vi "M9290A Configure Sweep.vi"(4 "Manual Mechanical Attenuation (10 dB)":dbl=10.0, 6 "Trigger Level":dbl=20.0, 7 "Trigger Source (0: Free Run)":i32(ring) items=["Free Run", "Video", "Line", "External1", "External2", "RF Burst"], 8 "error in":errorcluster, 9 "Span Frequency (50 kHz)":dbl, 10 "Center Frequency (100 MHz)":dbl=1000000000.0, 11 "VISA resource name":refnum<visa-resource-name>="SpecAn_1") -> (0 "error out":errorcluster)   [LabVIEW 2015]
uses:
  <instrlib>/Agilent MXA Series/Public/Configure/Configure Level (Normal).vi
  <instrlib>/Agilent MXA Series/Public/Configure/Trigger/Configure Trigger (Normal).vi
  <instrlib>/Agilent MXA Series/Public/Configure/Configure Frequency (Center Span).vi
  <instrlib>/Agilent MXA Series/Agilent MXA Series.lvlib
panel:
  out "VISA resource name out":refnum<visa-resource-name>
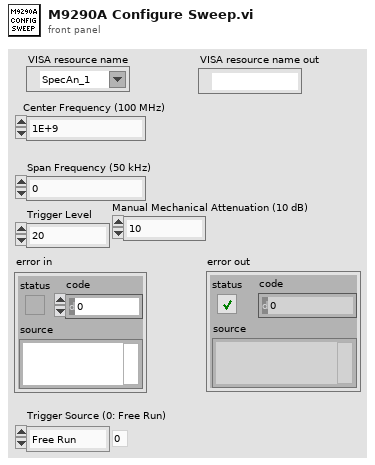
[diagram p1: front panel]
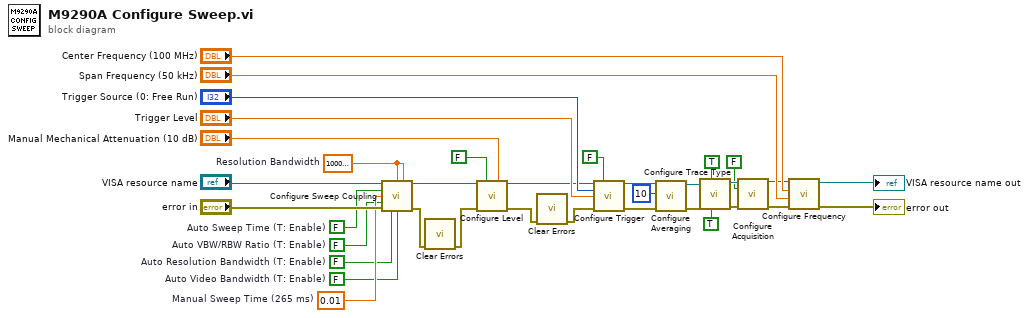
[diagram p0: block diagram]
diagram:
  w25 = 0.01  # Manual Sweep Time (265 ms)
  w14 = FALSE  # Auto VBW/RBW Ratio (T: Enable)
  w15 = FALSE  # Auto Video Bandwidth (T: Enable)
  w18 = FALSE  # Auto Sweep Time (T: Enable)
  w17 = FALSE  # Auto Resolution Bandwidth (T: Enable)
  w16 = 1000000.0  # Resolution Bandwidth
  n1 = call <instrlib>:"Configure Sweep Coupling.vi"("VISA resource name"="VISA resource name", "Manual Resolution Bandwidth (3E+6 Hz)"=w16, "Manual Video Bandwidth (3E+6 Hz)"=w16, "Auto Sweep Time (T: Enable)"=w18, "Manual Sweep Time (0.0663 s)"=w25, "Auto VBW/RBW Ratio (T: Enable)"=w14, "error in (no error)"="error in", "Auto Resolution Bandwidth (T: Enable)"=w17, "Auto Video Bandwidth (T: Enable)"=w15) -> ("VISA resource name out"=w7:refnum<visa-resource-name>, "error out"=w9:errorcluster)  [unwired: 5 in]
  n2 = call <vilib>:"Clear Errors.vi"("error in (no error)"=w9) -> ("error out"=w6:errorcluster)  [unwired: 5 in, 1 out]
  n3 = call-poly <instrlib>:"Configure Level.vi"("VISA resource name"=w7, "Auto Mechanical Attenuation (T: Enable)"=FALSE, "Manual Mechanical Attenuation (10 dB)"="Manual Mechanical Attenuation (10 dB)", "error in (no error)"=w6) -> ("VISA resource name out"=w5:refnum<visa-resource-name>, "error out"=w2:errorcluster)  [unwired: 10 in]
  n4 = call <vilib>:"Clear Errors.vi"("error in (no error)"=w2) -> ("error out"=w1:errorcluster)  [unwired: 5 in, 1 out]
  n5 = call-poly <instrlib>:"Configure Trigger.vi"("VISA resource name"=w5, "Enable Trigger Delay (F: Disable)"=FALSE ("Enable Trigger Delay (T: Enable)"), "Trigger Source (0: Free Run)"="Trigger Source (0: Free Run)", "Trigger Level (-20 dBm)"="Trigger Level", "error in (no error)"=w1) -> ("VISA resource name out"=w22:refnum<visa-resource-name>, "error out"=w12:errorcluster)  [unwired: 9 in]
  n6 = call <instrlib>:"Configure Averaging.vi"("error in (no error)"=w12, "Average Count (100)"=10, "VISA resource name"=w22) -> ("error out"=w20:errorcluster, "VISA resource name out"=w21:refnum<visa-resource-name>)  [unwired: 7 in]
  n7 = call <instrlib>:"Configure Trace Type.vi"("Enable Trace Display (F: Disable)"=TRUE, "Enable Trace Update (F: Disable)"=TRUE, "error in (no error)"=w20, "VISA resource name"=w21) -> ("error out"=w29:errorcluster, "VISA resource name out"=w30:refnum<visa-resource-name>)  [unwired: 6 in]
  n8 = call <instrlib>:"Configure Acquisition.vi"("VISA resource name"=w30, "Enable Continuous Sweep (T: Enable)"=FALSE, "error in (no error)"=w29) -> ("VISA resource name out"=w27:refnum<visa-resource-name>, "error out"=w26:errorcluster)  [unwired: 11 in]
  n9 = call-poly <instrlib>:"Configure Frequency.vi"("error in (no error)"=w26, "Span (2.65E+10 Hz)"="Span Frequency (50 kHz)", "Center Frequency (1.325E+10 Hz)"="Center Frequency (100 MHz)", "VISA resource name"=w27) -> ("error out"=→"error out":errorcluster, "VISA resource name out"=→"VISA resource name out":refnum<visa-resource-name>)  [unwired: 6 in]
